vi "GetMaxMinAvg.vi"(6 "calc cache":variant, 11 "waveform":waveform(sgl)) -> (2 "MaxMinAvg":T1, 4 "calc cache out":variant)   [LabVIEW 2017, in "AnalysisHelper.lvlib"]
uses:
  <vilib>/addons/InsightCM/Utilities/Analysis/Shared/AnalysisHelper.lvlib
  <vilib>/addons/InsightCM/Utilities/Analysis/Shared/controls/MaxMinAvgFeatures.ctl
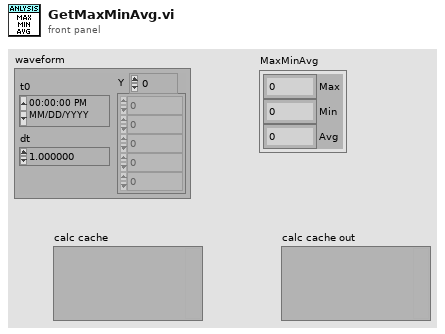
[diagram p1: front panel]
types:
  T1 = typedef "AnalysisHelper.lvlib/MaxMinAvgFeatures.ctl" = cluster{"Max":dbl, "Min":dbl, "Avg":dbl}
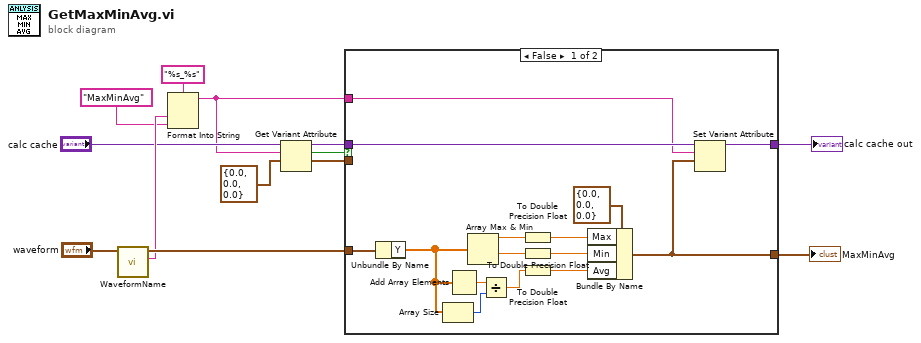
[diagram p0: block diagram]
diagram:
  n1 = call <vilib>:"WaveformName.vi"("signal in"="waveform") -> ("name"=w6:string, "signal out"=w8:waveform(sgl))  [unwired: 9 in]
  n2 = Format Into String(format string="%s_%s", w6, "MaxMinAvg" ("name")) -> (resulting string=w3:string)  [unwired: 2 in, 1 out]
  n3 = Get Variant Attribute(Variant="calc cache", name=w3, default value (empty Variant)=T1 {"Max"=0.0, "Min"=0.0, "Avg"=0.0} ("MaxMinAvg")) -> (duplicate Variant=w13:variant, found=w10:bool, value=w11:T1)  [unwired: 1 in, 1 out]
  n4 = case shown="False" w10 {
    tunnel: w8 -> [w18 _]
    tunnel: [w24 w30] -> w1
    tunnel: w13 -> [w25 w29]
    tunnel: w3 -> [w23 _]
    tunnel: [w22 w29] -> w12
    tunnel: w11 -> [_ w30]
    frame False {
      n5 = Unbundle By Name(w18) -> ("Y"=w15:sgl[])
      n6 = Array Size(array=w15) -> (size(s)=w16:i32)
      n7 = Add Array Elements(numeric array=w15) -> (sum=w17:sgl)
      n8 = Array Max & Min(array=w15) -> (max value=w20:sgl, min value=w19:sgl)  [unwired: 2 out]
      n9 = Divide(x=w17, y=w16) -> (x/y=w14:sgl)
      n10 = To Double Precision Float(number=w20) -> (double precision float=w28:dbl)
      n11 = To Double Precision Float(number=w19) -> (double precision float=w27:dbl)
      n12 = To Double Precision Float(number=w14) -> (double precision float=w26:dbl)
      n13 = Bundle By Name(cluster=T1 {"Max"=0.0, "Min"=0.0, "Avg"=0.0} ("MaxMinAvg"), "Max"=w28, "Min"=w27, "Avg"=w26) -> (w24:T1)
      n14 = Set Variant Attribute(Variant=w25, name=w23, value=w24) -> (Variant out=w22:variant)  [unwired: 1 in, 2 out]
    }
    frame True {
    }
  }
  "calc cache out" <- w12
  "MaxMinAvg" <- w1
